vi "Read Pulse Driver Configuration.vi"(8 "error in (no error)":errorcluster, 11 "Micron Optics Driver in":refnum<class "Micron Optics Driver.lvclass">) -> (0 "error out":errorcluster, 2 "Configuration":T1={"Post-trigger delay"=0.01, "Post-trigger duration"=0.1, "Rate"=1000000.0, "Ranges"=[10.0], "Re-name channels"=[], "Active channels"="0:1", "External clock"=FALSE} {"Rate" format="%#_8pHz"; "Post-trigger duration" format="%#_6ps"; "Post-trigger delay" format="%#_6ps"; "Ranges" format="%#_6pV"}, 3 "Micron Optics Driver out":refnum<class "Micron Optics Driver.lvclass">)   [LabVIEW 2024, in "Micron Optics Driver.lvclass"]
uses:
  Micron Optics Driver.lvclass
  Micron Optics Driver.lvclass/Micron Optics Driver.ctl
  Pulse Driver/Pusle Driver Configuration.ctl
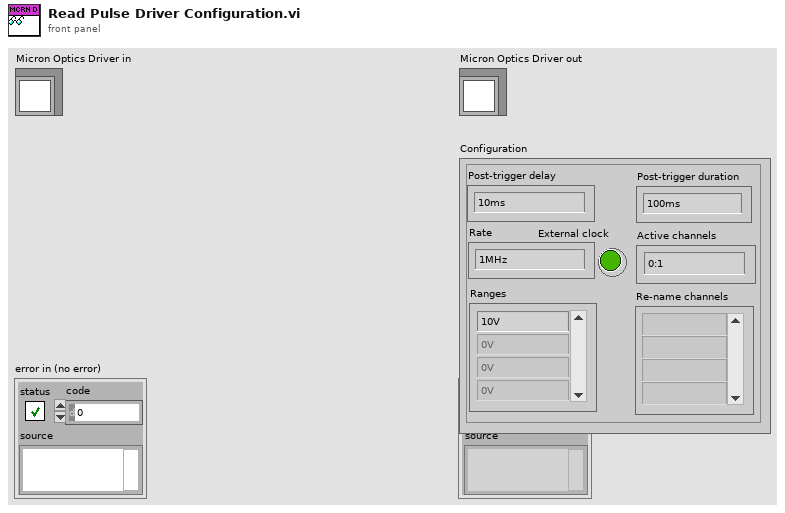
[diagram p1: front panel]
types:
  T1 = typedef "Pusle Driver Configuration.ctl" = cluster{"Post-trigger delay":dbl, "Post-trigger duration":dbl, "Rate":dbl, "Ranges":dbl[], "Re-name channels":string[], "Active channels":string, "External clock":bool}
  T2 = typedef "Micron optics didgitizer configuration.ctl" = cluster{"Post-trigger delay":dbl, "Post-trigger duration":dbl, "Rate":dbl, "Ranges":dbl[], "Re-name channels":string[], "Active channels":string, "External\nclock":bool, "Reference channel":i32, "Detection Setting IDs":u8[], "Stream and average":bool, "Address":string}
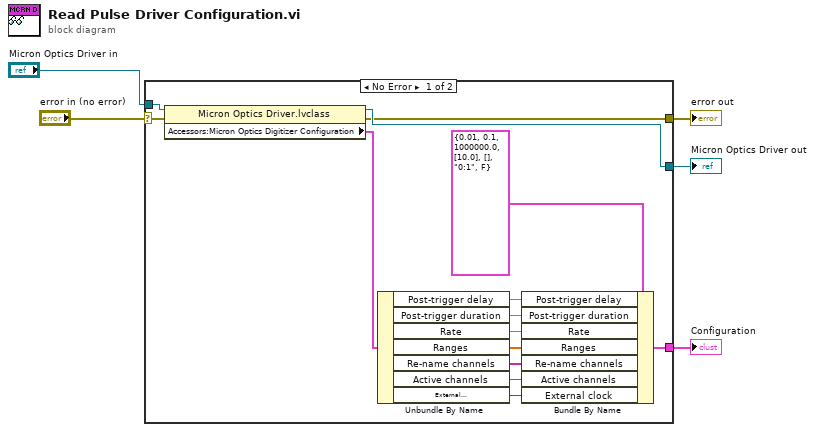
[diagram p0: block diagram]
diagram:
  n1 = case shown="No Error" "error in (no error)" {
    selector: "error in (no error)" -> [w10 w20]
    tunnel: [w11 w20] -> w4
    tunnel: [w12 w21] -> w2
    tunnel: "Micron Optics Driver in" -> [w13 w21]
    tunnel: [w9 _] -> w1
    frame No Error {
      n2 = property class="Micron Optics Driver.lvclass"(reference=w13, error in=w10) -> (reference out=w12:refnum<class "Micron Optics Driver.lvclass">, error out=w11:errorcluster, "Accessors:Micron Optics Digitizer Configuration"=w15:T2)
      n3 = Unbundle By Name(w15) -> ("Post-trigger delay"=w18:dbl, "Post-trigger duration"=w17:dbl, "Rate"=w16:dbl, "Ranges"=w19:dbl[], "Re-name channels"=w8:string[], "Active channels"=w7:string, "External\nclock"=w6:bool)
      n4 = Bundle By Name(cluster=T1 {"Post-trigger delay"=0.01, "Post-trigger duration"=0.1, "Rate"=1000000.0, "Ranges"=[10.0], "Re-name channels"=[], "Active channels"="0:1", "External clock"=FALSE} ("Pulse Driver Configuration"), "Post-trigger delay"=w18, "Post-trigger duration"=w17, "Rate"=w16, "Ranges"=w19, "Re-name channels"=w8, "Active channels"=w7, "External clock"=w6) -> (w9:T1)
    }
    frame Error {
    }
  }
  "error out" <- w4
  "Micron Optics Driver out" <- w2
  "Configuration" <- w1
